vi "get_measurements.vi"(0 "NInstrSim":refnum<class "NInstrSim.lvclass">, 5 "error in (no error)":errorcluster) -> (14 "dup NInstrSim":refnum<class "NInstrSim.lvclass">, 16 "dcMeasurement":dbl format="%_6g", 17 "waveform":waveform(dbl), 19 "error out":errorcluster)   [LabVIEW 2009, in "HB_Device_Examples.lvlib" / "NInstrSim.lvclass"]
uses:
  NInstrSim.lvclass
  NInstrSim.lvclass/NInstrSim.ctl
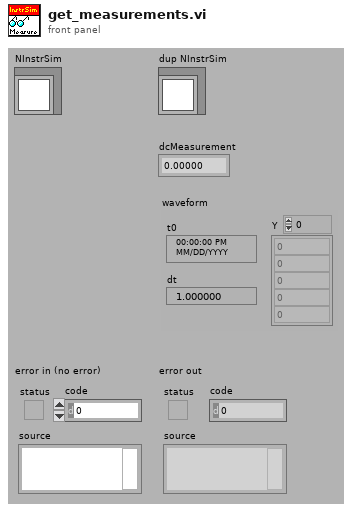
[diagram p1: front panel]
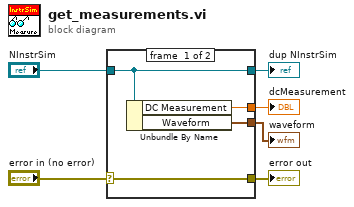
[diagram p0: block diagram]
diagram:
  n1 = case shown="No Error" "error in (no error)" {
    selector: "error in (no error)" -> [w10 w11]
    tunnel: [w10 w11] -> w5
    tunnel: [w9 w12] -> w3
    tunnel: "NInstrSim" -> [w9 w12]
    tunnel: [w8 _] -> w2
    tunnel: [w7 _] -> w1
    frame #0 {
      n2 = Unbundle By Name(w9) -> ("DC Measurement"=w8:dbl, "Waveform"=w7:waveform(dbl))
    }
    frame #1 {
    }
  }
  "error out" <- w5
  "dup NInstrSim" <- w3
  "dcMeasurement" <- w2
  "waveform" <- w1
